vi "Main.vi"() -> ()   [LabVIEW 2019, in "UPLINK.lvlib"]
doc: "This template is based off of the Queued Message Handler design pattern and the Queued Message Handler project template that ships with LabVIEW.\n\nThe main difference is that the queue is private to this module and communication between modules is performed via Broadcast and Request events.\n\nRequest events are wrapped in public API methods and are handled in the Event Handling Loop (EHL) of this VI. Any module can register for Broadcast events sent by this module. The EHL generates messages based on user interface actions.\n\nThe Message Handling Loop (MHL) processes messages generated by the EHL, or by other messages. The messages are string values, so new messages can be added easily to the Message Cases case structure in the MHL. Each message cluster can also provide an optional value for Message Data, which is a variant that can be converted to whatever message-specific data is required.\n_____\nBased on Delacor QMH Project Template 4.2.1.64."
uses:
  UPLINK.lvlib
  <vilib>/Delacor/Delacor QMH/Libraries/Module Admin_class/Delacor_lib_QMH_Module Admin.lvclass
  UI/Visual/Visual.xctl
  TypeDef/ISO.ctl
  Module Data--cluster.ctl
  Do Something Argument--cluster.ctl
  <vilib>/Delacor/Delacor QMH/Libraries/Message Queue_class/Delacor_lib_QMH_Message Queue.lvclass/Delacor_lib_QMH_Message Queue.ctl
  Do Something Else Argument--cluster.ctl
  Do Something Else and Wait for Reply Argument--cluster.ctl
  Do Something Else and Wait (Reply Payload)--cluster.ctl
  Stop Argument--cluster.ctl
  <vilib>/Delacor/Delacor QMH/Libraries/Module Admin_class/Delacor_lib_QMH_Module Admin.lvclass/Delacor_lib_QMH_Module Admin.ctl
  Ch_LINK Argument--cluster.ctl
  TypeDef/Sett data.ctl
  TypeDef/Noise.ctl
  TypeDef/Link.ctl
  Analys Argument--cluster.ctl
  TypeDef/Analys data.ctl
  TypeDef/Analys type.ctl
  <vilib>/Utility/miscctls.llb/LVPointTypeDef.ctl
  Class/ISO 14443 A UP.lvclass
  Class/ISO 14443 B UP.lvclass
  Class/Felica UP.lvclass
  Class/ISO 15693 UP.lvclass
  <vilib>/Delacor/Delacor QMH/Libraries/Message Queue_class/Delacor_lib_QMH_Enqueue Message (Single).vi
  <vilib>/Delacor/Delacor QMH/Libraries/Module Admin_class/Delacor_lib_QMH_Get External Launch.vi
  <vilib>/Utility/error.llb/Error Cluster From Error Code.vi
  <vilib>/ErrorRing/Error Ring.xnode
  <vilib>/Delacor/Delacor QMH/Libraries/Message Queue_class/Delacor_lib_QMH_Message Queue.lvclass
  Server/Server.lvlib
panel:
  out "ISO/IEC":T1
  out "Noise attenuator":dbl(knob) scale=0.0..10.0
  out "Q":dbl(slide) scale=0.0..10.0
  out "Visual":cluster{"Notes":string[], "Frame":u8[]}(xcontrol)
  in  "Simulate MHL Error":bool
  in  "Simulate EHL Error":bool
  out "error out":errorcluster
  in  "Module Admin":refnum<class "Delacor_lib_QMH_Module Admin.lvclass">
  out "X":dbl
  out "Status":string
  in  "Do Something Else <Replace Me>":bool
  in  "Do Something <Replace Me>":bool
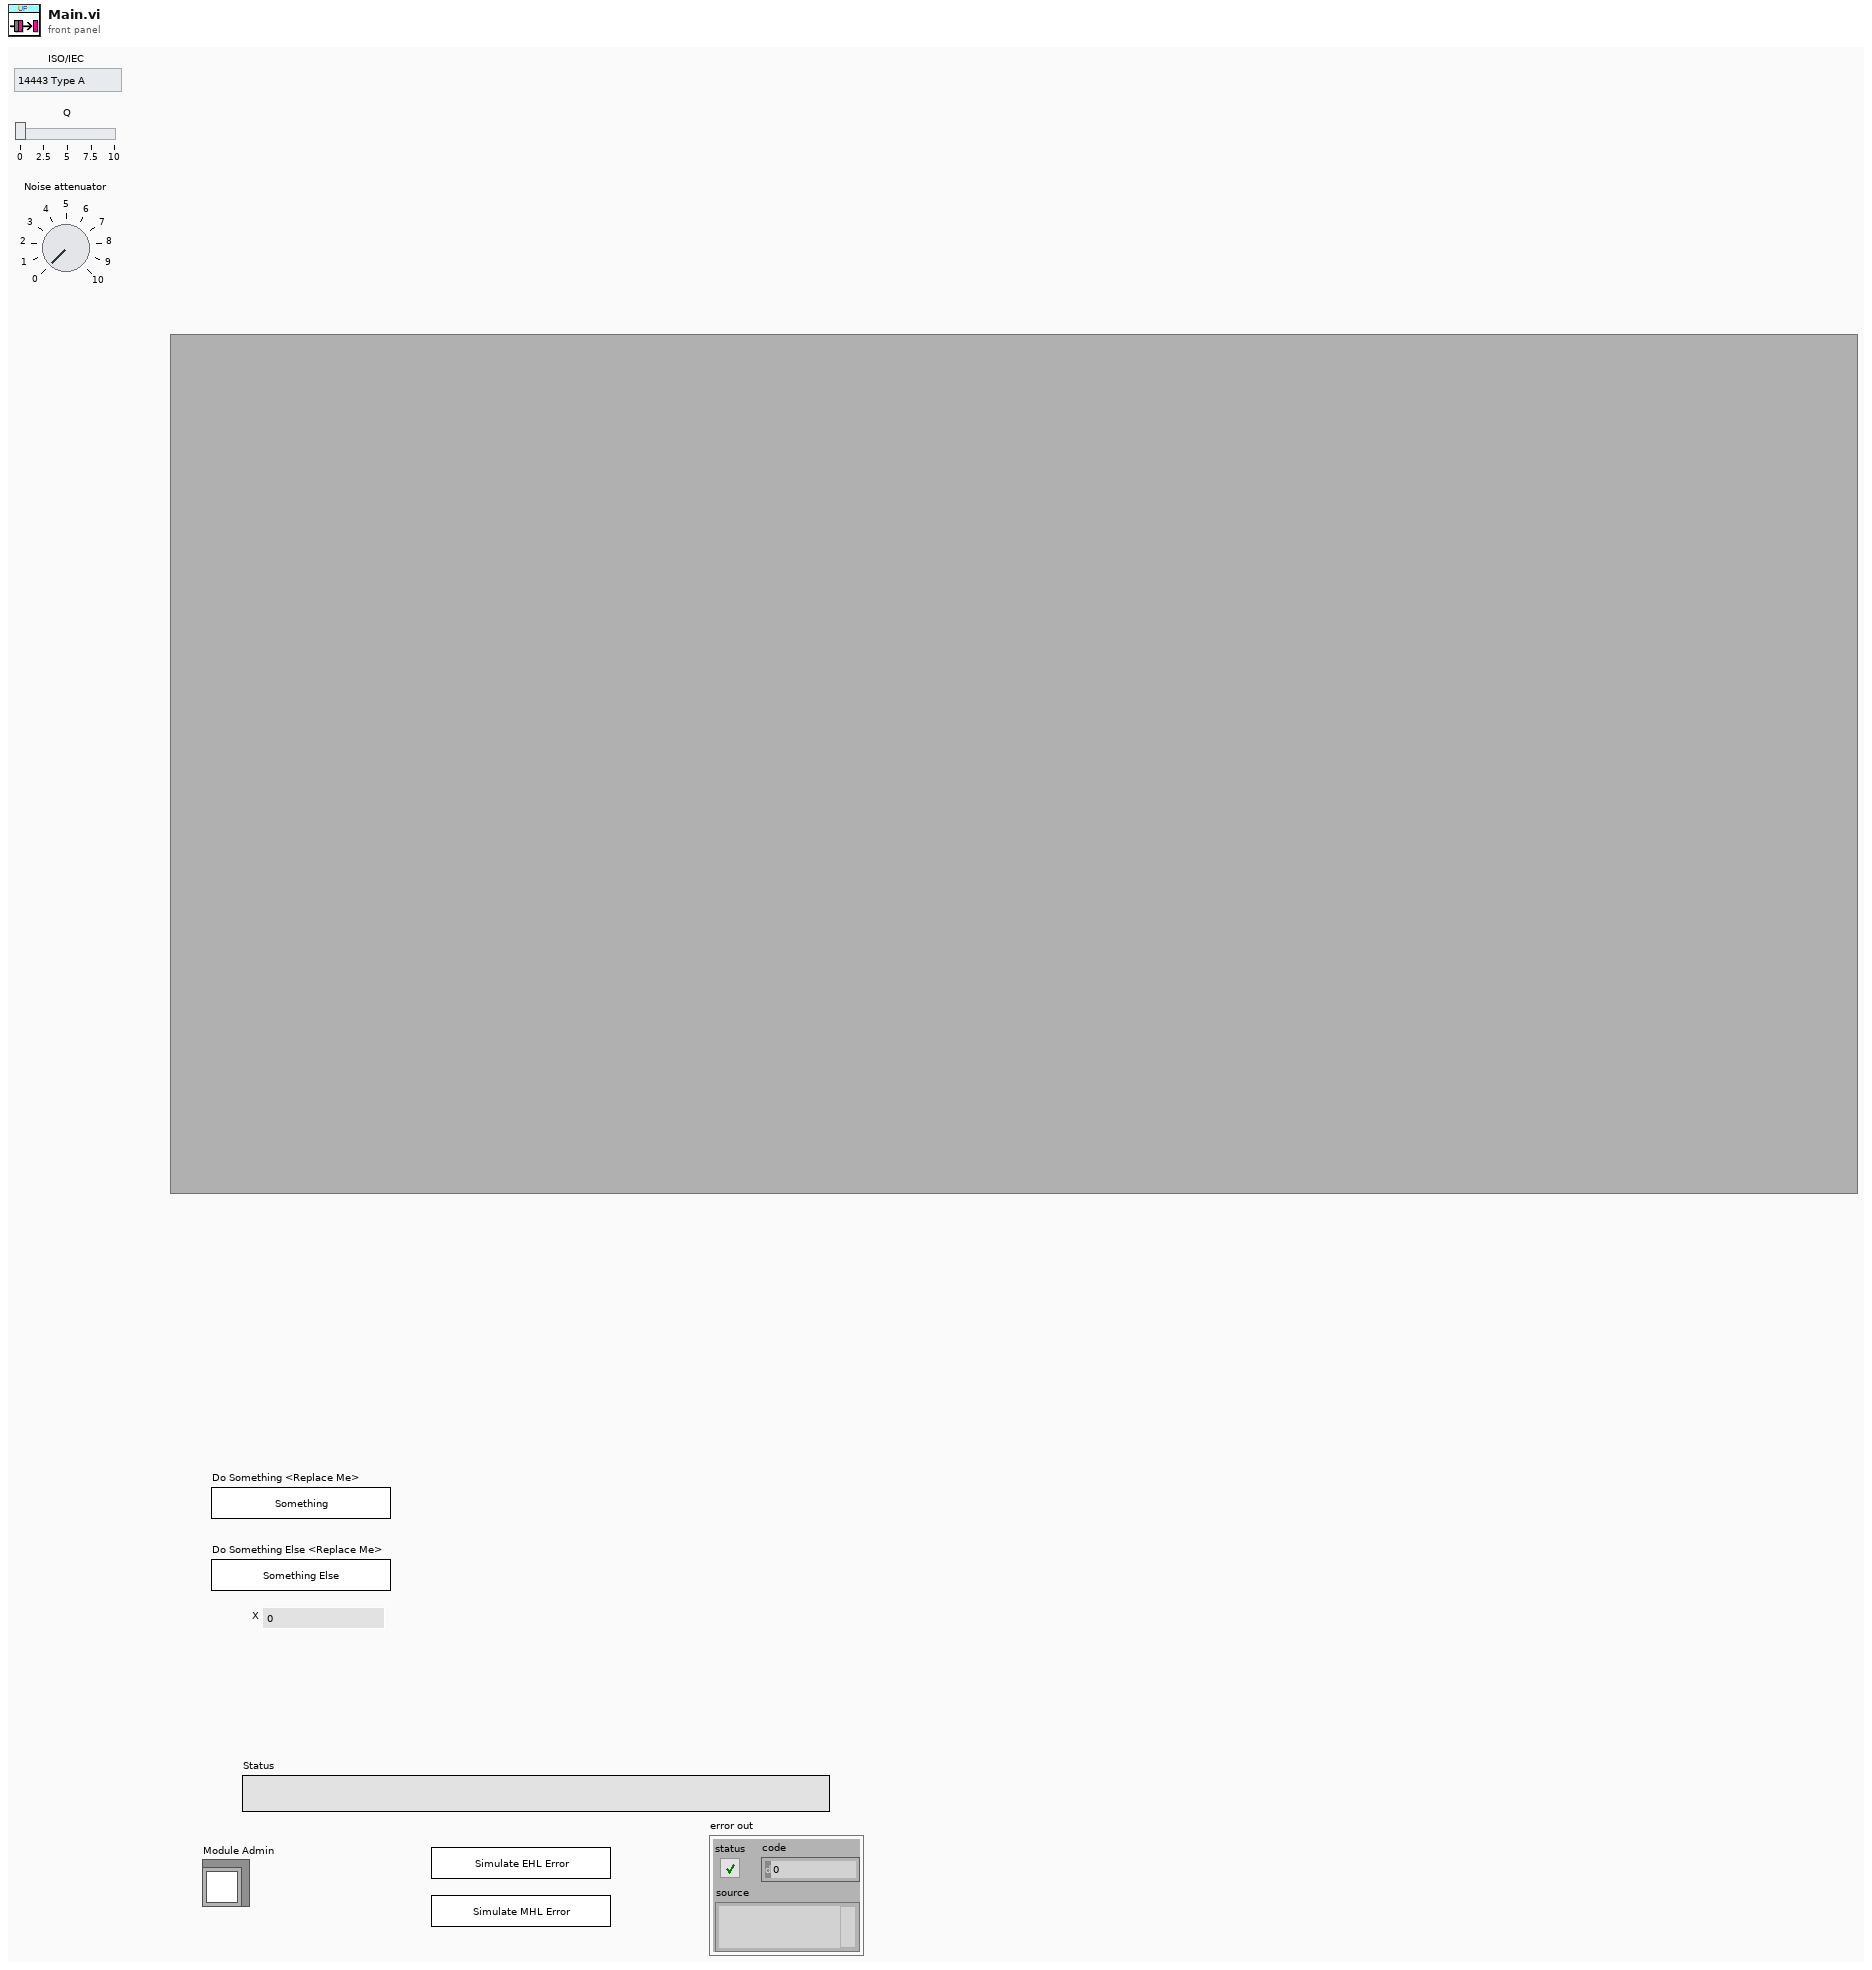
[diagram p1: front panel]
types:
  T1 = typedef "ISO.ctl" = enum16{"14443 Type A", "14443 Type B", "Felica", "15693"}
  T2 = typedef "UPLINK.lvlib/Request Events--cluster.ctl" = cluster{"Stop Module":refnum<user-event>, "Do Something":refnum<user-event>, "Do Something Else":refnum<user-event>, "Do Something Else and Wait for Reply":refnum<user-event>, "Show Panel":refnum<user-event>, "Hide Panel":refnum<user-event>, "Get Module Execution Status":refnum<user-event>, "Show Diagram":refnum<user-event>, "Ch_LINK":refnum<user-event>, "Analys":refnum<user-event>}
  T3 = typedef "Server.lvlib/Broadcast Events--cluster.ctl" = cluster{"Module Did Init":refnum<user-event>, "Status Updated":refnum<user-event>, "Error Reported":refnum<user-event>, "Did Something":refnum<user-event>, "Module Did Stop":refnum<user-event>, "Update Module Execution Status":refnum<user-event>, "Apply settings":refnum<user-event>}
  T4 = typedef "UPLINK.lvlib/Module Data--cluster.ctl" = cluster{"Status":string}
  T5 = typedef "UPLINK.lvlib/Do Something Argument--cluster.ctl" = cluster{"Do Something Msg":string}
  T6 = typedef "UPLINK.lvlib/Do Something Else Argument--cluster.ctl" = cluster{"Do Something Else Msg":string, "X":dbl}
  T7 = typedef "UPLINK.lvlib/Do Something Else and Wait for Reply Argument--cluster.ctl" = cluster{"Do Something Else Msg":string, "X":dbl, "Wait Notifier":refnum<notifier>, "wait for reply":bool}
  T8 = enum32{"invalid lock state", "Not Locked", "Locked (No Password)", "Password-protected"}
  T9 = typedef "UPLINK.lvlib/Stop Argument--cluster.ctl" = cluster{"Origin":string, "Exit via Stop Module Req?":bool, "Wait for Module to stop?":bool}
  T10 = typedef "UPLINK.lvlib/Ch_LINK Argument--cluster.ctl" = cluster{"Subpanel Ref":refnum<vi>}
  T11 = typedef "Link.ctl" = enum16{"UPLINK", "DOWNLINK"}
  T12 = typedef "Sett data.ctl" = cluster{"Filter":i32, "Gain":dbl, "Bit rate":dbl, "ISO/IEC w ":T1, "BI":cluster{"R":dbl, "C":dbl, "L":dbl}, "BM":cluster{"R":dbl, "C":dbl, "L":dbl}, "M":cluster{"Метка":i64, "Считыветель":i64}, "Type noise":T13, "Link":T11, "Noise attenuator":dbl, "Signal gain":dbl, "Distance":dbl}
  T13 = typedef "Noise.ctl" = enum16{"Гауссовский шум", "Белый шум"}
  T14 = typedef "UPLINK.lvlib/Analys Argument--cluster.ctl" = cluster{"data":T15, "Data link":variant}
  T15 = typedef "Analys data.ctl" = cluster{"min attenuator":dbl, "max distanse":dbl, "num sample":dbl, "type":T16}
  T16 = typedef "Analys type.ctl" = enum16{"Noise", "Distance"}
  T17 = typedef "LVPointTypeDef.ctl" = cluster{"Horizontal":i16, "Vertical":i16}
  T18 = enum32{"Invalid", "Standard", "Closed", "Hidden", "Minimized", "Maximized"}
  T19 = typedef "UPLINK.lvlib/Do Something Else and Wait (Reply Payload)--cluster.ctl" = cluster{"Value":dbl, "error":errorcluster}
  T20 = typedef "Visual.xctl/data.ctl" = cluster{"Notes":string[], "Frame":u8[]}
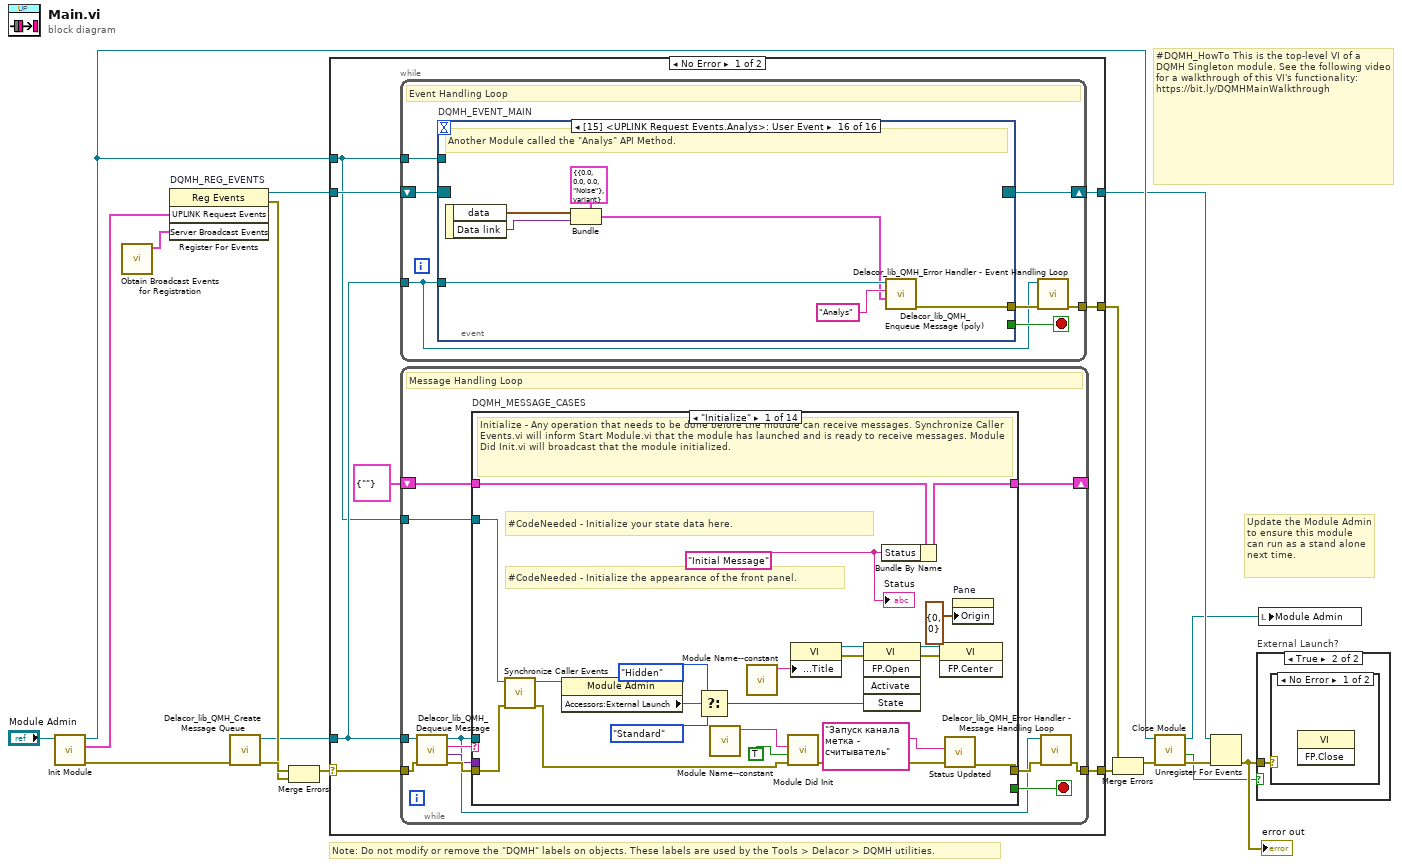
[diagram p0: block diagram]
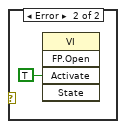
[diagram p3: hidden frame]
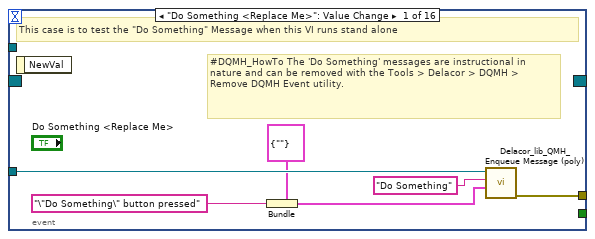
[diagram p4: hidden frame]
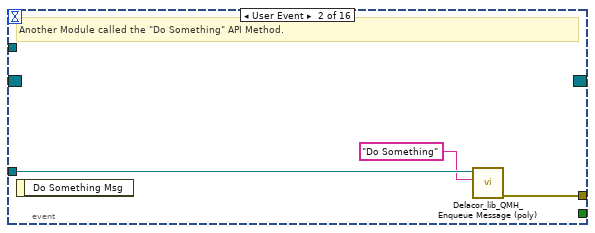
[diagram p5: hidden frame]
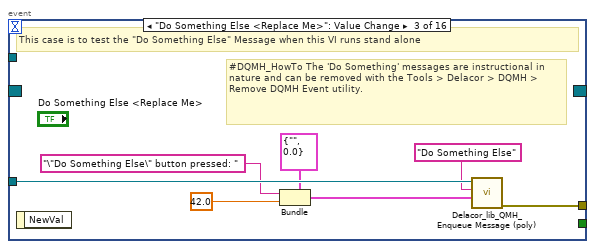
[diagram p6: hidden frame]
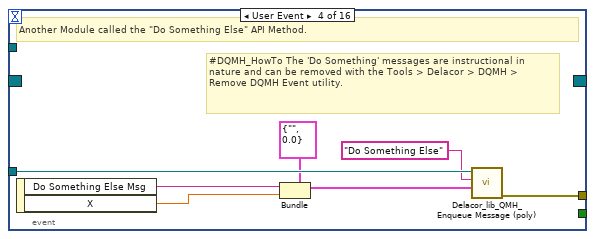
[diagram p7: hidden frame]
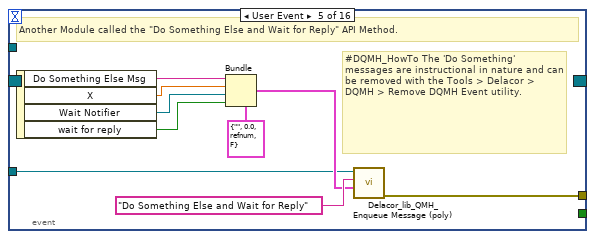
[diagram p8: hidden frame]
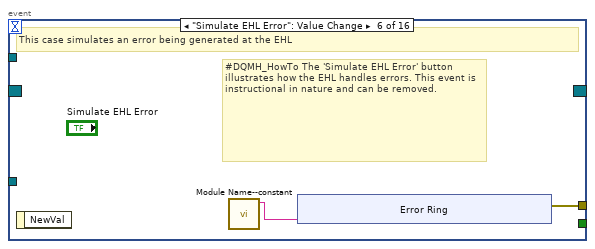
[diagram p9: hidden frame]
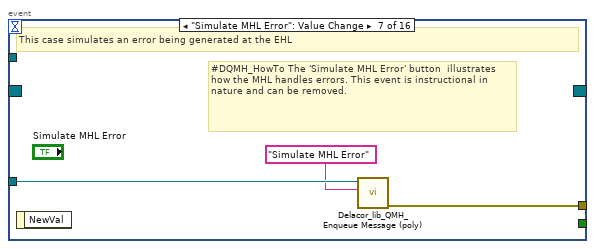
[diagram p10: hidden frame]
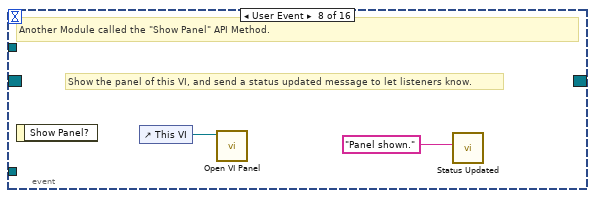
[diagram p11: hidden frame]
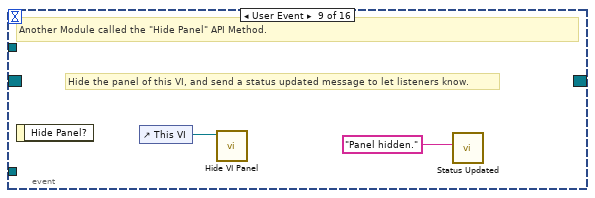
[diagram p12: hidden frame]
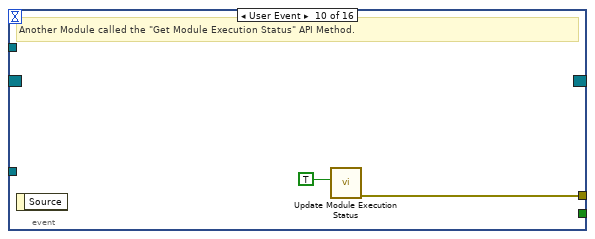
[diagram p13: hidden frame]
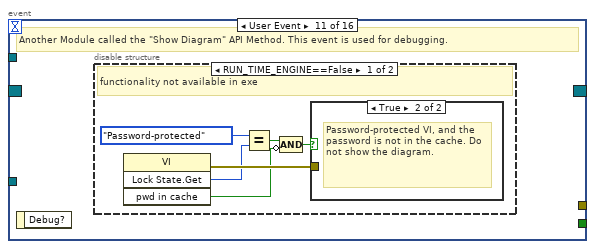
[diagram p14: hidden frame]
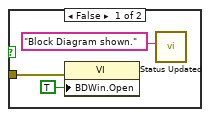
[diagram p15: hidden frame]
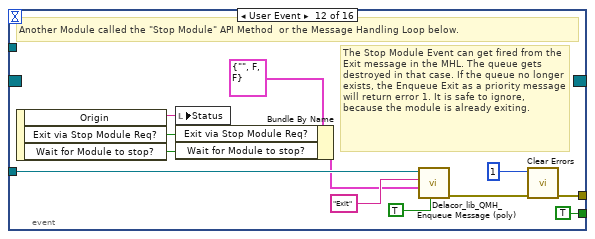
[diagram p17: hidden frame]
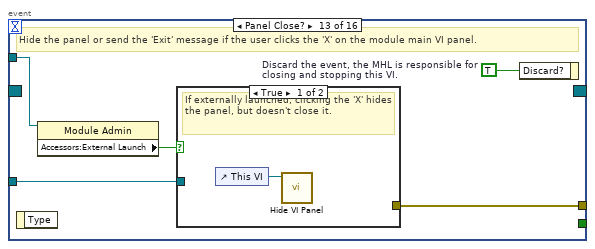
[diagram p18: hidden frame]
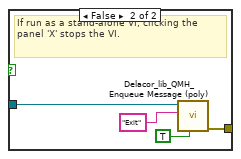
[diagram p19: hidden frame]
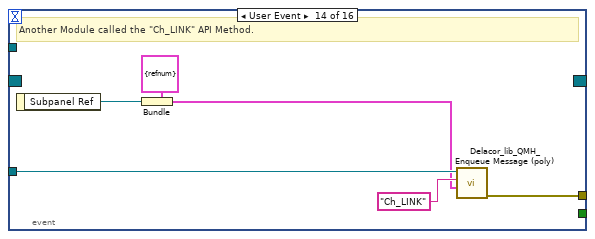
[diagram p20: hidden frame]
diagram:
  # "#DQMH_HowTo This is the top-level VI of a DQMH Singleton module. See the following video for a walkthrough of this VI's functionality: https://bit.ly/DQMHMainWalkthrough"
  # "Note: Do not modify or remove the \"DQMH\" labels on objects. These labels are used by the Tools > Delacor > DQMH utilities."
  # "Update the Module Admin to ensure this module can run as a stand alone next time."
  n1 = call "Init Module.vi"("Singleton Module Admin in"="Module Admin") -> ("error out"=w17:errorcluster, "UPLINK Request Events"=w6:T2, "Singleton Module Admin out"=w9:refnum<class "Delacor_lib_QMH_Module Admin.lvclass">)  [unwired: 8 in]
  n2 = call "Obtain Broadcast Events for Registration.vi"() -> ("Server Broadcast Events"=w1:T3)  [unwired: 9 in, 2 out]
  n3 = register-events "DQMH_REG_EVENTS"(w6, w1) -> (reference out=w7:refnum<event-registration>, error out=w10:errorcluster)  [unwired: 2 in]
  n4 = call <vilib>:"Delacor_lib_QMH_Create Message Queue.vi"("error in (no error)"=w17) -> ("error out"=w12:errorcluster, "Message Queue"=w5:refnum<class "Delacor_lib_QMH_Message Queue.lvclass">)  [unwired: 9 in]
  n5 = Merge Errors(w12, w10) -> (w11:errorcluster)
  n6 = case shown="No Error" w11 {
    selector: w11 -> [w24 w341]
    tunnel: [w26 w341] -> w18
    tunnel: [w23 w338] -> w8
    tunnel: w7 -> [w21 w338]
    tunnel: w5 -> [w20 _]
    tunnel: [w25 _] -> w15
    tunnel: w9 -> [w19 w334]
    frame No Error {
      n7 = while {
        tunnel: w20 -> [w27]
        shift-right: [w30] -> w23
        shift-left: w21 -> [w31]
        tunnel: [w32] -> w25
        tunnel: w19 -> [w28]
        stop <- w29 stop-if-true
        # "Event Handling Loop"
        n8 = event "DQMH_EVENT_MAIN" shown="[15] <UPLINK Request Events.Analys>: User Event" {
          selector: w31 -> [_ _ _ _ _ _ _ _ _ _ _ _ _ _ _ _]
          dyn-events: [_ _ _ _ _ _ _ _ _ _ _ _ _ _ _ _] -> w30
          timeout: _ -> [_ _ _ _ _ _ _ _ _ _ _ _ _ _ _ _]
          tunnel: [_ _ _ _ _ _ _ _ _ _ _ TRUE ("Discard?") _ _ _ _] -> w29
          tunnel: w27 -> [w38 w41 w48 w55 w58 _ w76 _ _ _ _ w100 w107 w120 w121 w142]
          tunnel: [w39 w42 w49 w56 w65 w67 w77 _ _ w83 _ w103 w109 w115 w124 w137] -> w33
          tunnel: w28 -> [_ _ _ _ _ _ _ _ _ _ _ _ w106 _ _ _]
          event "Do Something <Replace Me>": Value Change {
            # "#DQMH_HowTo The 'Do Something' messages are instructional in nature and can be removed with the Tools > Delacor > DQMH > Remove DQMH Event utility."
            # "This case is to test the \"Do Something\" Message when this VI runs stand alone"
            n9 = event-data() -> ()  [unwired: 1 in, 1 out]
            n10 = Bundle(cluster=T5 {"Do Something Msg"=""} ("Do Something Argument"), "Do Something Msg"="\"Do Something\" button pressed" ("\"Do Something\" button pressed")) -> (w34:T5)
            n11 = call-poly <vilib>:"Delacor_lib_QMH_Enqueue Message (poly).vi"("Message Data"=w34, "Message"="Do Something", "Message Queue in"=w38) -> ("error out"=w39:errorcluster)  [unwired: 7 in, 1 out]
          }
          event User Event {
            # "Another Module called the \"Do Something\" API Method."
            n12 = event-data() -> ()  [unwired: 1 in, 1 out]
            n13 = call-poly <vilib>:"Delacor_lib_QMH_Enqueue Message (poly).vi"("Message"="Do Something", "Message Queue in"=w41) -> ("error out"=w42:errorcluster)  [unwired: 8 in, 1 out]
          }
          event "Do Something Else <Replace Me>": Value Change {
            # "#DQMH_HowTo The 'Do Something' messages are instructional in nature and can be removed with the Tools > Delacor > DQMH > Remove DQMH Event utility."
            # "This case is to test the \"Do Something Else\" Message when this VI runs stand alone"
            n14 = event-data() -> ()  [unwired: 1 in, 1 out]
            n15 = Bundle(cluster=T6 {"Do Something Else Msg"="", "X"=0.0} ("Do Something Else Argument"), "Do Something Else Msg"="\"Do Something Else\" button pressed: " ("\"Do Something Else\" button pressed"), "X"=42.0) -> (w45:T6)
            n16 = call-poly <vilib>:"Delacor_lib_QMH_Enqueue Message (poly).vi"("Message Data"=w45, "Message"="Do Something Else", "Message Queue in"=w48) -> ("error out"=w49:errorcluster)  [unwired: 7 in, 1 out]
          }
          event User Event {
            # "#DQMH_HowTo The 'Do Something' messages are instructional in nature and can be removed with the Tools > Delacor > DQMH > Remove DQMH Event utility."
            # "Another Module called the \"Do Something Else\" API Method."
            n17 = event-data() -> ("Do Something Else Msg"=w51:string, "X"=w50:dbl)  [unwired: 1 in]
            n18 = Bundle(cluster=T6 {"Do Something Else Msg"="", "X"=0.0} ("Do Something Else Argument"), "Do Something Else Msg"=w51, "X"=w50) -> (w52:T6)
            n19 = call-poly <vilib>:"Delacor_lib_QMH_Enqueue Message (poly).vi"("Message Data"=w52, "Message"="Do Something Else", "Message Queue in"=w55) -> ("error out"=w56:errorcluster)  [unwired: 7 in, 1 out]
          }
          event User Event {
            # "#DQMH_HowTo The 'Do Something' messages are instructional in nature and can be removed with the Tools > Delacor > DQMH > Remove DQMH Event utility."
            # "Another Module called the \"Do Something Else and Wait for Reply\" API Method."
            n20 = event-data() -> ("Do Something Else Msg"=w61:string, "X"=w60:dbl, "Wait Notifier"=w59:refnum<notifier>, "wait for reply"=w57:bool)  [unwired: 1 in]
            n21 = Bundle(cluster=T7 {"Do Something Else Msg"="", "X"=0.0, "Wait Notifier"=refnum, "wait for reply"=FALSE} ("Do Something Else and Wait for Reply Argument"), "Do Something Else Msg"=w61, "X"=w60, "Wait Notifier"=w59, "wait for reply"=w57) -> (w62:T7)
            n22 = call-poly <vilib>:"Delacor_lib_QMH_Enqueue Message (poly).vi"("Message Data"=w62, "Message"="Do Something Else and Wait for Reply", "Message Queue in"=w58) -> ("error out"=w65:errorcluster)  [unwired: 7 in, 1 out]
          }
          event "Simulate EHL Error": Value Change {
            # "#DQMH_HowTo The 'Simulate EHL Error' button  illustrates how the EHL handles errors. This event is instructional in nature and can be removed."
            # "This case simulates an error being generated at the EHL"
            n23 = event-data() -> ()  [unwired: 1 in, 1 out]
            n24 = call "Module Name--constant.vi"() -> ("Module Name"=w66:string)  [unwired: 11 in]
            n25 = xnode "Error Ring"("parameter 0"=w66) -> ("error out"=w67:errorcluster)
          }
          event "Simulate MHL Error": Value Change {
            # "#DQMH_HowTo The 'Simulate MHL Error' button  illustrates how the MHL handles errors. This event is instructional in nature and can be removed."
            # "This case simulates an error being generated at the EHL"
            n26 = event-data() -> ()  [unwired: 1 in, 1 out]
            n27 = call-poly <vilib>:"Delacor_lib_QMH_Enqueue Message (poly).vi"("Message"="Simulate MHL Error", "Message Queue in"=w76) -> ("error out"=w77:errorcluster)  [unwired: 8 in, 1 out]
          }
          event User Event {
            # "Show the panel of this VI, and send a status updated message to let listeners know."
            # "Another Module called the \"Show Panel\" API Method."
            n28 = event-data() -> ()  [unwired: 1 in, 1 out]
            n29 = control-ref of="This VI"() -> (w79:refnum<vi>)
            n30 = call "Open VI Panel.vi"("VI"=w79) -> ()  [unwired: 10 in, 1 out]
            n31 = call "Status Updated.vi"("Status"="Panel shown." ("format string")) -> ()  [unwired: 10 in, 1 out]
          }
          event User Event {
            # "Hide the panel of this VI, and send a status updated message to let listeners know."
            # "Another Module called the \"Hide Panel\" API Method."
            n32 = event-data() -> ()  [unwired: 1 in, 1 out]
            n33 = control-ref of="This VI"() -> (w81:refnum<vi>)
            n34 = call "Hide VI Panel.vi"("VI"=w81) -> ()  [unwired: 10 in, 1 out]
            n35 = call "Status Updated.vi"("Status"="Panel hidden." ("format string")) -> ()  [unwired: 10 in, 1 out]
          }
          event User Event {
            # "Another Module called the \"Get Module Execution Status\" API Method."
            n36 = event-data() -> ()  [unwired: 1 in, 1 out]
            n37 = call "Update Module Execution Status.vi"("Running?"=TRUE) -> ("error out"=w83:errorcluster)  [unwired: 10 in]
          }
          event User Event {
            # "Another Module called the \"Show Diagram\" API Method. This event is used for debugging."
            n38 = event-data() -> ()  [unwired: 1 in, 1 out]
            n39 = disable-structure shown="RUN_TIME_ENGINE==False" {
              frame condition #0 (active) {
                # "functionality not available in exe"
                n40 = invoke class="VI" method="Lock State.Get"() -> (error out=w89:errorcluster, "Get Lock State"=w88:T8, "pwd in cache"=w85:bool)  [unwired: 4 in, 1 out]
                n41 = Equal?(x=T8."Password-protected", y=w88) -> (x = y?=w86:bool)
                n42 = Compound Arithmetic op=AND(w86, invert w85) -> (w84:bool)
                n43 = case shown="True" w84 {
                  tunnel: w89 -> [w92 _]
                  frame False {
                    n44 = property class="VI"(error in=w92, "BDWin.Open"=TRUE ("Block Diagram Window:Open")) -> ()  [unwired: 1 in, 2 out]
                    n45 = call "Status Updated.vi"("Status"="Block Diagram shown." ("format string")) -> ()  [unwired: 10 in, 1 out]
                  }
                  frame True {
                    # "Password-protected VI, and the password is not in the cache. Do not show the diagram."
                  }
                }
              }
              frame condition #1 {
              }
            }
          }
          event User Event {
            # "The Stop Module Event can get fired from the Exit message in the MHL. The queue gets destroyed in that case. If the queue no longer exists, the Enqueue Exit as a priority message will return error 1. It is safe to ignore, because the module is already exiting."
            # "Another Module called the \"Stop Module\" API Method  or the Message Handling Loop below."
            n46 = event-data() -> ("Origin"=w99:string, "Exit via Stop Module Req?"=w95:bool, "Wait for Module to stop?"=w94:bool)  [unwired: 1 in]
            n47 = local write "Status"(w99) -> ()
            n48 = Bundle By Name(cluster=T9 {"Origin"="", "Exit via Stop Module Req?"=FALSE, "Wait for Module to stop?"=FALSE} ("Stop Argument"), "Exit via Stop Module Req?"=w95, "Wait for Module to stop?"=w94) -> (w93:T9)
            n49 = call-poly <vilib>:"Delacor_lib_QMH_Enqueue Message (poly).vi"("Priority Message? (F)"=TRUE, "Message Data"=w93, "Message"="Exit", "Message Queue in"=w100) -> ("error out"=w104:errorcluster)  [unwired: 6 in, 1 out]
            n50 = call <vilib>:"Clear Errors.vi"("error in (no error)"=w104, "specific error code to clear (0: all)"=1) -> ("error out"=w103:errorcluster)  [unwired: 4 in, 1 out]
          }
          event Panel Close? {
            w108 = TRUE  # Discard the event, the MHL is responsible for closing and stopping this VI.
            # "Hide the panel or send the 'Exit' message if the user clicks the 'X' on the module main VI panel."
            n51 = event-data() -> ()  [unwired: 1 in, 1 out]
            n52 = property class="Module Admin"(reference=w106) -> ("Accessors:External Launch"=w105:bool)  [unwired: 1 in, 2 out]
            n53 = case shown="True" w105 {
              tunnel: w107 -> [_ w113]
              tunnel: [_ w114] -> w109
              frame True {
                # "If externally launched, clicking the 'X' hides the panel, but doesn't close it."
                n54 = control-ref of="This VI"() -> (w110:refnum<vi>)
                n55 = call "Hide VI Panel.vi"("VI"=w110) -> ()  [unwired: 10 in, 1 out]
              }
              frame False {
                # "If run as a stand-alone VI, clicking the panel 'X' stops the VI."
                n56 = call-poly <vilib>:"Delacor_lib_QMH_Enqueue Message (poly).vi"("Priority Message? (F)"=TRUE, "Message"="Exit", "Message Queue in"=w113) -> ("error out"=w114:errorcluster)  [unwired: 7 in, 1 out]
              }
            }
            n57 = event-data("Discard?"=w108) -> ()  [unwired: 1 in, 1 out]
          }
          event User Event {
            # "Another Module called the \"Ch_LINK\" API Method."
            n58 = event-data() -> ("Subpanel Ref"=w116:refnum<vi>)  [unwired: 1 in]
            n59 = Bundle(cluster=T10 {"Subpanel Ref"=refnum} ("Ch_LINK Argument"), "Subpanel Ref"=w116) -> (w117:T10)
            n60 = call-poly <vilib>:"Delacor_lib_QMH_Enqueue Message (poly).vi"("Message Data"=w117, "Message"="Ch_LINK", "Message Queue in"=w120) -> ("error out"=w115:errorcluster)  [unwired: 7 in, 1 out]
          }
          event User Event {
            n61 = event-data() -> ("Data"=w122:variant)  [unwired: 1 in, 4 out]
            n62 = Variant To Data(type=T12 {"Filter"=0, "Gain"=0.0, "Bit rate"=0.0, "ISO/IEC w "=enum."14443 Type A", "BI"={"R"=0.0, "C"=0.0, "L"=0.0}, "BM"={"R"=0.0, "C"=0.0, "L"=0.0}, "M"={"Метка"=4, "Считыветель"=4}, "Type noise"=enum."Гауссовский шум", "Link"=enum."UPLINK", "Noise attenuator"=0.0, "Signal gain"=1.0, "Distance"=0.0} ("Sett data"), Variant=w122) -> (data=w123:T12, error out=w129:errorcluster)  [unwired: 1 in]
            n63 = Unbundle By Name(w123) -> ("Link"=w127:T11)
            n64 = Equal?(x=w127, y=Link."UPLINK" ("Link")) -> (x = y?=w125:bool)
            n65 = case shown="True" w125 {
              tunnel: w129 -> [w130 w135]
              tunnel: [w130 w133] -> w124
              tunnel: w122 -> [_ w132]
              tunnel: w121 -> [_ w131]
              frame False {
              }
              frame True {
                n66 = call-poly <vilib>:"Delacor_lib_QMH_Enqueue Message (poly).vi"("error in (no error)"=w135, "Message Data"=w132, "Message"="UPLINK", "Message Queue in"=w131) -> ("error out"=w133:errorcluster)  [unwired: 6 in, 1 out]
              }
            }
          }
          event User Event {
            # "Another Module called the \"Analys\" API Method."
            n67 = event-data() -> ("data"=w138:T15, "Data link"=w136:variant)  [unwired: 1 in]
            n68 = Bundle(cluster=T14 {"data"={"min attenuator"=0.0, "max distanse"=0.0, "num sample"=0.0, "type"=enum."Noise"}, "Data link"=variant} ("Analys Argument"), "data"=w138, "Data link"=w136) -> (w139:T14)
            n69 = call-poly <vilib>:"Delacor_lib_QMH_Enqueue Message (poly).vi"("Message Data"=w139, "Message"="Analys", "Message Queue in"=w142) -> ("error out"=w137:errorcluster)  [unwired: 7 in, 1 out]
          }
        }
        n70 = call-dynamic "Delacor_lib_QMH_Error Handler - Event Handling Loop.vi"("error in (no error)"=w33, "Message Queue in"=w27) -> ("dup error in"=w32:errorcluster)  [unwired: 8 in, 1 out]
      }
      n71 = while {
        tunnel: w20 -> [w145]
        shift-right: [w149] -> _
        shift-left: T4 {"Status"=""} ("Data Cluster") -> [w150]
        tunnel: w24 -> [w153]
        tunnel: [w151] -> w26
        tunnel: w19 -> [w143]
        stop <- w148 stop-if-true
        # "Message Handling Loop"
        n72 = call-dynamic "Delacor_lib_QMH_Dequeue Message.vi"("error in (no error)"=w153, "Message Queue in"=w145) -> ("error out"=w152:errorcluster, "Message Data"=w146:variant, "Message"=w147:string, "Message Queue out"=w144:refnum<class "Delacor_lib_QMH_Message Queue.lvclass">)  [unwired: 6 in]
        n73 = case "DQMH_MESSAGE_CASES" shown="\"Initialize\"" w147 {
          selector: w147 -> [_ _ _ _ _ _ _ _ _ _ _ _ _ w321]
          tunnel: w144 -> [_ _ _ _ _ _ _ _ _ _ _ w290 w313 _]
          tunnel: w152 -> [w174 w178 w186 w195 w214 w236 w251 w270 w273 w275 w280 w297 w319 w323]
          tunnel: [w157 w178 w184 w194 w213 w234 w238 w258 w272 w275 w279 w293 w316 w324] -> w154
          tunnel: w150 -> [w165 w177 w183 w193 w211 w235 w252 w269 w271 w274 w277 w292 w312 w322]
          tunnel: [w164 w177 w183 w193 w211 w235 w252 w269 w271 w274 w277 w292 w312 w322] -> w149
          tunnel: [_ _ _ _ _ _ _ _ _ _ _ _ w311 _] -> w148
          tunnel: w146 -> [_ _ w182 w190 w208 w233 w250 w268 _ _ _ w291 w310 _]
          tunnel: w143 -> [w166 _ _ _ _ _ _ _ _ _ _ w289 w305 _]
          frame "Initialize" {
            w159 = "Initial Message" ("Initial Message")
            # "#CodeNeeded - Initialize the appearance of the front panel."
            # "#CodeNeeded - Initialize your state data here."
            # "Initialize - Any operation that needs to be done before the module can receive messages. Synchronize Caller Events.vi will inform Start Module.vi that the module has launched and is ready to receive messages. Module Did Init.vi will broadcast that the module initialized."
            n74 = call "Synchronize Caller Events.vi"("error in (no error)"=w174, "Singleton Module Admin in"=w166) -> ("error out"=w155:errorcluster, "Singleton Module Admin out"=w161:refnum<class "Delacor_lib_QMH_Module Admin.lvclass">)  [unwired: 8 in]
            n75 = property class="Module Admin"(reference=w161) -> ("Accessors:External Launch"=w170:bool)  [unwired: 1 in, 2 out]
            n76 = Select(t=T18."Hidden" ("State"), s=w170, f=T18."Standard" ("State")) -> (s? t:f=w167:T18)
            n77 = call "Module Name--constant.vi"() -> ("Module Name"=w162:string)  [unwired: 11 in]
            n78 = call "Module Name--constant.vi"() -> ("Module Name"=w173:string)  [unwired: 11 in]
            n79 = call "Module Did Init.vi"("error in (no error)"=w155, "Initialized?"=TRUE, "Origin"=w162) -> ("error out"=w158:errorcluster)  [unwired: 8 in]
            n80 = property class="VI"("Front Panel.Title"=w173) -> (reference out=w172:refnum<vi>, error out=w176:errorcluster)  [unwired: 2 in]
            n81 = invoke class="VI" method="FP.Open"(reference=w172, error in=w176, "State"=w167) -> (reference out=w171:refnum<vi>, error out=w175:errorcluster)  [unwired: 2 in, 3 out]
            n82 = Bundle By Name(cluster=w165, "Status"=w159) -> (w164:T4)
            n83 = invoke class="VI" method="FP.Center"(reference=w171, error in=w175) -> ()  [unwired: 1 in, 3 out]
            n84 = call "Status Updated.vi"("error in (no error)"=w158, "Status"="Запуск канала метка - считыватель") -> ("error out"=w157:errorcluster)  [unwired: 9 in]
            n85 = property on="Pane" class="Pane"("Origin"=T17 {"Horizontal"=0, "Vertical"=0}) -> ()  [unwired: 2 in, 2 out]
            "Status" <- w159
          }
          frame "--- Module Specific ---" {
            # "Separator -- The following cases handle messages specific to this Module."
          }
          frame "Do Something" {
            # "#DQMH_HowTo The 'Do Something' messages are instructional in nature and can be removed with the Tools > Delacor > DQMH > Remove DQMH Event utility."
            # "Do Something - Replace this message with functionality for your own application. Note that this message also fires the \"Did Something\" broadcast event."
            n86 = Variant To Data(error in=w186, type=T5 {"Do Something Msg"=""} ("Do Something Argument"), Variant=w182) -> (data=w181:T5, error out=w185:errorcluster)
            n87 = Unbundle By Name(w181) -> ("Do Something Msg"=w179:string)
            n88 = call "Did Something.vi"("error in (no error)"=w185, "Did Something Msg"=w179) -> ("error out"=w184:errorcluster)  [unwired: 9 in]
            n89 = local write "Status"(w179) -> ()
            n90 = call "Status Updated.vi"("Status"=w179) -> ()  [unwired: 10 in, 1 out]
          }
          frame "Do Something Else" {
            # "#DQMH_HowTo The 'Do Something' messages are instructional in nature and can be removed with the Tools > Delacor > DQMH > Remove DQMH Event utility."
            # "Do Something Else - Replace this message with functionality for your own application."
            n91 = Variant To Data(error in=w195, type=T6 {"Do Something Else Msg"="", "X"=0.0} ("Do Something Else Argument"), Variant=w190) -> (data=w191:T6, error out=w194:errorcluster)
            n92 = Unbundle By Name(w191) -> ("Do Something Else Msg"=w189:string, "X"=w188:dbl)
            "X" <- w188
            n93 = Format Into String(initial string=w189, w188) -> (resulting string=w187:string)  [unwired: 2 in, 1 out]
            n94 = local write "Status"(w187) -> ()
            n95 = call "Status Updated.vi"("Status"=w187) -> ()  [unwired: 10 in, 1 out]
          }
          frame "Do Something Else and Wait for Reply" {
            w203 = "X(%.2f)+Offset(%.2f)=%.2f"  # status message format string
            # "#DQMH_HowTo The 'Do Something' messages are instructional in nature and can be removed."
            # "Send back X with a random offset"
            # "Do Something Else and Wait for Reply - Replace this message with functionality for your own application. Note that this message must fire a notifier to let callers know it has finished execution, and it returns an error if the 'Value' is negative."
            n96 = Random Number (0-1)() -> (number: 0 to 1=w205:dbl)
            n97 = Variant To Data(error in=w214, type=T7 {"Do Something Else Msg"="", "X"=0.0, "Wait Notifier"=refnum, "wait for reply"=FALSE} ("Do Something Else and Wait for Reply Argument"), Variant=w208) -> (data=w209:T7, error out=w212:errorcluster)
            n98 = Unbundle By Name(w209) -> ("Wait Notifier"=w196:refnum<notifier>, "Do Something Else Msg"=w207:string, "X"=w204:dbl, "wait for reply"=w200:bool)
            n99 = Add(x=w205, y=w204) -> (x+y=w199:dbl)
            n100 = local write "X"(w204) -> ()
            n101 = Less Than 0?(x=w199) -> (x < 0?=w202:bool)
            n102 = Format Into String(format string=w203, initial string=w207, w204, w205, w199) -> (resulting string=w201:string)  [unwired: 1 in, 1 out]
            n103 = case shown="True" w202 {
              tunnel: [_ w221] -> w197
              frame False {
              }
              frame True {
                n104 = xnode "Error Ring"() -> ("error out"=w221:errorcluster)
              }
            }
            n105 = Bundle By Name(cluster=T19 {"Value"=0.0, "error"={"status"=FALSE, "code"=0, "source"=""}} ("notification"), "error"=w197, "Value"=w199) -> (w198:T19)
            n106 = local write "Status"(w201) -> ()
            n107 = call "Status Updated.vi"("Status"=w201) -> ()  [unwired: 10 in, 1 out]
            n108 = case shown="False" w200 {
              tunnel: w198 -> [_ w217]
              tunnel: w196 -> [_ w216]
              frame False {
              }
              frame True {
                # "Simulate an operation that requires a wait."
                n109 = flat-sequence {
                  tunnel: w217 -> [w220]
                  tunnel: w216 -> [w219]
                  tunnel: w215 -> [_]
                  frame #0 {
                    n110 = Send Notification(notification=w220, notifier=w219) -> ()  [unwired: 1 in, 2 out]
                  }
                }
                n111 = Wait (ms)(milliseconds to wait=u32 1000) -> (millisecond timer value=w215:u32)
              }
            }
            n112 = Merge Errors(w212, w197) -> (w213:errorcluster)
          }
          frame "Ch_LINK" {
            # "#CodeNeeded\n1. Configure this Message Case for handling the \"Ch_LINK\" message.\n2. Delete or edit this label when done."
            # "Change link on server VI"
            n113 = Variant To Data(error in=w236, type=T10 {"Subpanel Ref"=refnum} ("Ch_LINK Argument"), Variant=w233) -> (data=w231:T10, error out=w234:errorcluster)
            n114 = Unbundle By Name(w231) -> ("Subpanel Ref"=w228:refnum<vi>)
            n115 = call "Module Name--constant.vi"() -> ("Module Name"=w227:string)  [unwired: 11 in]
            n116 = property class="VI"("Front Panel.Title"=w227) -> (reference out=w229:refnum<vi>, error out=w230:errorcluster)  [unwired: 2 in]
            n117 = call "Insert SubPanel.vi"("error in (no error)"=w230, "VI Ref"=w229, "Subpanel Ref"=w228) -> ()  [unwired: 8 in, 1 out]
          }
          frame "UPLINK" {
            n118 = Variant To Data(error in=w251, type=T12 {"Filter"=0, "Gain"=0.0, "Bit rate"=0.0, "ISO/IEC w "=enum."14443 Type A", "BI"={"R"=0.0, "C"=0.0, "L"=0.0}, "BM"={"R"=0.0, "C"=0.0, "L"=0.0}, "M"={"Метка"=4, "Считыветель"=4}, "Type noise"=enum."Гауссовский шум", "Link"=enum."UPLINK", "Noise attenuator"=0.0, "Signal gain"=1.0, "Distance"=0.0} ("Sett data"), Variant=w250) -> (data=w242:T12, error out=w237:errorcluster)
            n119 = Unbundle By Name(w242) -> ("ISO/IEC w"=w247:T1)
            n120 = call "Start load.vi"("error in (no error)"=w237) -> ("error out"=w240:errorcluster)  [unwired: 10 in]
            n121 = case shown="\"15693\"" w247 {
              tunnel: [refnum<class "ISO 14443 A UP.lvclass"> refnum ("ISO 14443 A UP.lvclass") refnum<class "ISO 14443 B UP.lvclass"> refnum ("ISO 14443 B UP.lvclass") refnum<class "Felica UP.lvclass"> refnum ("Felica UP.lvclass") refnum<class "ISO 15693 UP.lvclass"> refnum ("ISO 15693 UP.lvclass")] -> w249
              frame "14443 Type A", Default {
              }
              frame "14443 Type B" {
              }
              frame "Felica" {
              }
              frame "15693" {
              }
            }
            n122 = call "OOP_UP.vi"("error in (no error)"=w240, "Sett data"=w242, "RFID system in"=w249) -> ("error out"=w245:errorcluster, "Error on  byte"=w243:dbl, "Visual"=→"Visual":T20)  [unwired: 6 in]
            n123 = Format Into String(format string="Произведен расчет канала.\nВероятность ошибки на бит составляет: %#.3f", w243) -> (resulting string=w244:string)  [unwired: 2 in, 1 out]
            n124 = call "Status Updated.vi"("error in (no error)"=w245, "Status"=w244) -> ("error out"=w239:errorcluster)  [unwired: 9 in]
            n125 = call "Stop load.vi"("error in (no error)"=w239) -> ("error out"=w238:errorcluster)  [unwired: 10 in]
          }
          frame "Analys" {
            # "Do analys of error on bit"
            n126 = Variant To Data(error in=w270, type=T14 {"data"={"min attenuator"=0.0, "max distanse"=0.0, "num sample"=0.0, "type"=enum."Noise"}, "Data link"=variant} ("Analys Argument"), Variant=w268) -> (data=w266:T14, error out=w257:errorcluster)
            n127 = call "Start load.vi"("error in (no error)"=w257) -> ("error out"=w259:errorcluster)  [unwired: 10 in]
            n128 = call "Status Updated.vi"("error in (no error)"=w259, "Status"="Запуск анализа") -> ("error out"=w264:errorcluster)  [unwired: 9 in]
            n129 = call "Analys UP.vi"("error in"=w264, "data"=w266) -> ("error out"=w262:errorcluster, "output cluster"=w265:cluster{"Array":dbl[], "Array":dbl[]})  [unwired: 8 in]
            n130 = call "Analys Chart.vi"("error in (no error)"=w262, "error wave in"=w265) -> ()  [unwired: 3 in]
            n131 = call "Status Updated.vi"("error in (no error)"=w262, "Status"="Окончание анализа") -> ("error out"=w260:errorcluster)  [unwired: 9 in]
            n132 = call "Stop load.vi"("error in (no error)"=w260) -> ("error out"=w258:errorcluster)  [unwired: 10 in]
          }
          frame "---Copy This Frame---" {
            # "Duplicate this frame when creating new messages.  Change this comment in the duplicated frame to describe this message."
            n133 = Merge Errors(w273) -> (w272:errorcluster)
          }
          frame "--- Exit and Error Handling---" {
            # "Separator - The following cases handle errors and exit messages."
          }
          frame "Simulate MHL Error" {
            # "#DQMH_HowTo The 'Simulate MHL Error' button  illustrates how the MHL handles errors. This event is instructional in nature and can be removed."
            # "Simulate an error occurring at the MHL"
            n134 = call "Module Name--constant.vi"() -> ("Module Name"=w276:string)  [unwired: 11 in]
            n135 = xnode "Error Ring"("parameter 0"=w276) -> ("error out"=w278:errorcluster)
            n136 = Merge Errors(w280, w278) -> (w279:errorcluster)
          }
          frame "Error" {
            # "#CodeRecommended - If you ever change the name of this \"Error\" message, you'll need to update the name in the Check Loop Error.vi as well."
            # "#CodeRecommended - If the module is running in standalone mode (External Launch = FALSE), this code will pop up an error dialog and call the 'Exit' message if an error occurs. Add more fine-grained error handling here."
            # "Error - Check the error message data and respond accordingly. This message is sent by the \"Error Handler\" VIs at the end of each loop in this application."
            n137 = property class="Module Admin"(reference=w289) -> ("Accessors:External Launch"=w288:bool)  [unwired: 1 in, 2 out]
            n138 = Variant To Data(error in=w297, type=errorcluster {"status"=FALSE, "code"=0, "source"=""} ("error constant"), Variant=w291) -> (data=w298:errorcluster, error out=w295:errorcluster)
            n139 = call "Error Reported.vi"("Error"=w298) -> ()  [unwired: 10 in, 1 out]
            n140 = case shown="False" w288 {
              tunnel: [w303 _] -> w294
              tunnel: w290 -> [w301 _]
              tunnel: w298 -> [w302 _]
              frame False {
                # "If the module is running standalone, then pop up an error dialog and call the \"Exit\" message."
                n141 = call <vilib>:"Simple Error Handler.vi"("error in (no error)"=w302) -> ()  [unwired: 4 in, 5 out]
                n142 = call-poly <vilib>:"Delacor_lib_QMH_Enqueue Message (poly).vi"("Priority Message? (F)"=TRUE, "Message"="Exit", "Message Queue in"=w301) -> ("error out"=w303:errorcluster)  [unwired: 7 in, 1 out]
              }
              frame True {
                # "If the module was launched externally, calling the Error Reported broadcast VI is the only action performed by the \"Error\" message. The module's caller can then process the error appropriately."
              }
            }
            n143 = Merge Errors(w295, w294) -> (w293:errorcluster)
            n144 = local write "error out"(w293) -> ()
          }
          frame "Exit" {
            w309 = 91  # 91: not all Exit messages will have an argument
            w311 = TRUE  # Stop the VI
            # "Release the message queue reference"
            # "Exit - Exit the application."
            n145 = Variant To Data(error in=w319, type=T9 {"Origin"="", "Exit via Stop Module Req?"=FALSE, "Wait for Module to stop?"=FALSE} ("Stop Argument"), Variant=w310) -> (data=w307:T9, error out=w315:errorcluster)
            n146 = call <vilib>:"Clear Errors.vi"("error in (no error)"=w315, "specific error code to clear (0: all)"=w309) -> ("error out"=w318:errorcluster)  [unwired: 4 in, 1 out]
            n147 = call "Status Updated.vi"("Status"="Остановка канала метка - считыватель") -> ()  [unwired: 10 in, 1 out]
            n148 = control-ref of="This VI"() -> (w306:refnum<vi>)
            n149 = call-dynamic "Delacor_lib_QMH_Release Message Queue.vi"("error in (no error)"=w318, "Message Queue"=w313) -> ("error out"=w317:errorcluster)  [unwired: 9 in]
            n150 = call "Handle Exit.vi"("Stop Argument"=w307, "Admin in"=w305, "VI reference"=w306) -> ("error out"=w314:errorcluster)  [unwired: 7 in, 1 out]
            n151 = Merge Errors(w317, w314) -> (w316:errorcluster)
          }
          frame Default {
            # "'Default' case only runs if there is a message that isn't defined in any of the other cases.  Output a programming error."
            n152 = call "Module Name--constant.vi"() -> ("Module Name"=w320:string)  [unwired: 11 in]
            n153 = xnode "Error Ring"("parameter 0"=w321, "parameter 1"=w320) -> ("error out"=w325:errorcluster)
            n154 = Merge Errors(w323, w325) -> (w324:errorcluster)
          }
        }
        n155 = call-dynamic "Delacor_lib_QMH_Error Handler - Message Handling Loop.vi"("error in (no error)"=w154, "Message Queue in"=w144) -> ("dup error in"=w151:errorcluster)  [unwired: 8 in, 1 out]
      }
    }
    frame Error {
      # "Synchronize Caller Events.vi will inform Start Module.vi that the module has launched and will let the code calling Start Module.vi register for broadcasts and would permit the caller receive the broadcast that an error occurred at launch time."
      n156 = call "Synchronize Caller Events.vi"("Singleton Module Admin in"=w334) -> ("error out"=w339:errorcluster)  [unwired: 9 in, 1 out]
      n157 = call "Module Name--constant.vi"() -> ("Module Name"=w337:string)  [unwired: 11 in]
      n158 = Format Into String(format string="An error occurred during initialization. %s is no longer running.", w337) -> (resulting string=w335:string)  [unwired: 2 in, 1 out]
      n159 = Merge Errors(w341, w339) -> (w340:errorcluster)
      n160 = call "Error Reported.vi"("Additional Information"=w335, "Error"=w340) -> ()  [unwired: 9 in, 1 out]
    }
  }
  n161 = Merge Errors(w15, w18) -> (w14:errorcluster)
  n162 = call "Close Module.vi"("error in (no error)"=w14, "Module Admin in"=w9) -> ("error out"=w16:errorcluster, "External Launch"=w2:bool, "Module Admin out"=w3:refnum<class "Delacor_lib_QMH_Module Admin.lvclass">)  [unwired: 7 in]
  n163 = Unregister For Events(event registration refnum=w8, error in=w16) -> (error out=w13:errorcluster)
  "error out" <- w13
  n164 = case "External Launch?" shown="True" w2 {
    tunnel: w13 -> [_ w342]
    frame False {
    }
    frame True {
      n165 = case shown="No Error" w342 {
        frame No Error {
          n166 = invoke class="VI" method="FP.Close"() -> ()  [unwired: 3 in, 3 out]
        }
        frame Error {
          n167 = invoke class="VI" method="FP.Open"("Activate"=TRUE ("Activate?")) -> ()  [unwired: 4 in, 5 out]
        }
      }
    }
  }
  n168 = local write "Module Admin"(w3) -> ()
